vi "OEE_create_queues.vi"(8 "error_in":errorcluster, 11 "all_config_info_in":T1={"main_ini_file"={"SQL Driver"="", "SQL Server"="", "SQL Database"="", "SQL UID"="", "Reference table"="", "Reference history"="", "Archivisation CFG table"="", "Archivisation CFG history"="", "User table"="", "User history"="", "Default reference"="", "Update pulse[ms]"=0, "default language"="", "SCREEN 1 Left"=0, "SCREEN 1 Top"=10, "SCREEN 1 Width"=0, "SCREEN 1 Height"=0, "SCREEN 2 Left"=0, "SCREEN 2 Top"=0, "SCREEN 2 Width"=0, "SCREEN 2 Height"=10}, "SQL Password"="", "queue_refnums"={"MAIN_queue"=refnum, "SCREEN_1_queue"=refnum, "SCREEN_2_queue"=refnum, "PULSE_queue"=refnum, "GRAPH_TOGGLE_queue"=refnum}}) -> (0 "error_out":errorcluster, 3 "all_config_info_out":T1={"main_ini_file"={"SQL Driver"="", "SQL Server"="", "SQL Database"="", "SQL UID"="", "Reference table"="", "Reference history"="", "Archivisation CFG table"="", "Archivisation CFG history"="", "User table"="", "User history"="", "Default reference"="", "Update pulse[ms]"=0, "default language"="", "SCREEN 1 Left"=0, "SCREEN 1 Top"=10, "SCREEN 1 Width"=0, "SCREEN 1 Height"=0, "SCREEN 2 Left"=0, "SCREEN 2 Top"=0, "SCREEN 2 Width"=0, "SCREEN 2 Height"=10}, "SQL Password"="", "queue_refnums"={"MAIN_queue"=refnum, "SCREEN_1_queue"=refnum, "SCREEN_2_queue"=refnum, "PULSE_queue"=refnum, "GRAPH_TOGGLE_queue"=refnum}})   [LabVIEW 2019]
uses:
  ini/typedef/OEE_all_config_info.ctl
  ini/typedef/OEE_main_ini_file.ctl
  typedef/OEE_queue_refnums.ctl
  typedef/OEE_MAIN_queue_element.ctl
  MAIN/OEE_MAIN_sequence_state.ctl
  typedef/OEE_SCREEN_1_queue_element.ctl
  SCREEN_1/OEE_SCREEN_1_sequence_state.ctl
  typedef/OEE_SCREEN_2_queue_element.ctl
  SCREEN_2/OEE_SCREEN_2_sequence_state.ctl
  typedef/OEE_PULSE_queue_element.ctl
  PULSE/OEE_PULSE_sequence_state.ctl
  typedef/OEE_GRAPH_TOGGLE_TIMER_queue_element.ctl
  SCREEN_2/GRAPH_TOGGLE_TIMER/OEE_GRAPH_TOGGLE_TIMER_sequence_state.ctl
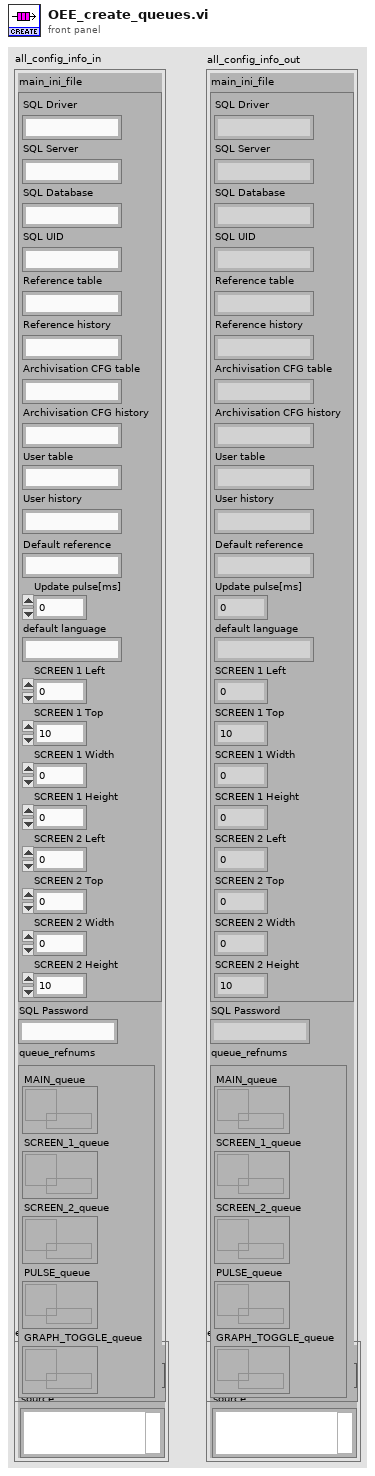
[diagram p1: front panel]
types:
  T1 = typedef "OEE_all_config_info.ctl" = cluster{"main_ini_file":T2, "SQL Password":string, "queue_refnums":T3}
  T2 = typedef "OEE_main_ini_file.ctl" = cluster{"SQL Driver":string, "SQL Server":string, "SQL Database":string, "SQL UID":string, "Reference table":string, "Reference history":string, "Archivisation CFG table":string, "Archivisation CFG history":string, "User table":string, "User history":string, "Default reference":string, "Update pulse[ms]":i32, "default language":string, "SCREEN 1 Left":i16, "SCREEN 1 Top":i16, "SCREEN 1 Width":i16, "SCREEN 1 Height":i16, "SCREEN 2 Left":i16, "SCREEN 2 Top":i16, "SCREEN 2 Width":i16, "SCREEN 2 Height":i16}
  T3 = typedef "OEE_queue_refnums.ctl" = cluster{"MAIN_queue":refnum<queue>, "SCREEN_1_queue":refnum<queue>, "SCREEN_2_queue":refnum<queue>, "PULSE_queue":refnum<queue>, "GRAPH_TOGGLE_queue":refnum<queue>}
  T4 = typedef "OEE_GRAPH_TOGGLE_TIMER_queue_element.ctl" = cluster{"state":T5, "variable":variant}
  T5 = typedef "OEE_GRAPH_TOGGLE_TIMER_sequence_state.ctl" = enum16{"initialize", "get_next_state", "start_toggling", "stop_toggling", "do_toggle", "error", "stop"}
  T6 = typedef "OEE_PULSE_queue_element.ctl" = cluster{"state":T7, "variable":variant}
  T7 = typedef "OEE_PULSE_sequence_state.ctl" = enum16{"initialize", "get_next_state", "start_pulses", "stop_pulses", "pulse", "error", "stop"}
  T8 = typedef "OEE_MAIN_queue_element.ctl" = cluster{"state":T9, "variable":variant}
  T9 = typedef "OEE_MAIN_sequence_state.ctl" = enum16{"initialize", "get_next_state", "get_SQL_data", "update_displays", "error", "stop"}
  T10 = typedef "OEE_SCREEN_2_queue_element.ctl" = cluster{"state":T11, "variable":variant}
  T11 = typedef "OEE_SCREEN_2_sequence_state.ctl" = enum16{"initialize", "get_next_state", "update", "show", "hide", "error", "stop"}
  T12 = typedef "OEE_SCREEN_1_queue_element.ctl" = cluster{"state":T13, "variable":variant}
  T13 = typedef "OEE_SCREEN_1_sequence_state.ctl" = enum16{"initialize", "get_next_state", "update", "show", "hide", "error", "stop"}
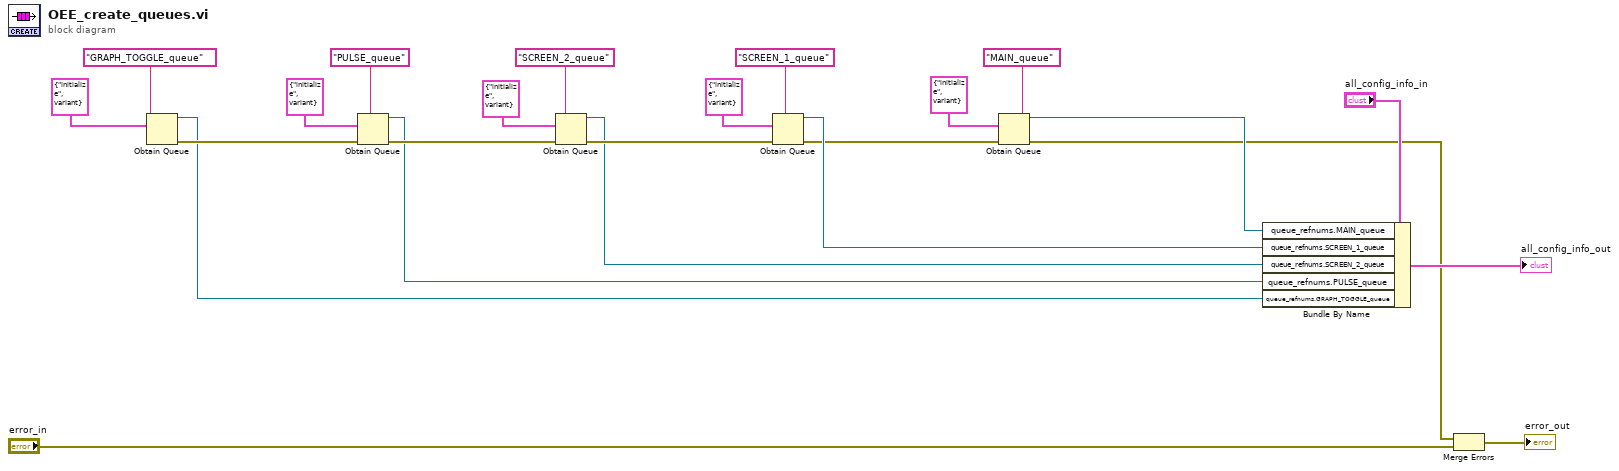
[diagram p0: block diagram]
diagram:
  n1 = Obtain Queue(name (unnamed)="GRAPH_TOGGLE_queue", element data type=T4 {"state"=enum."initialize", "variable"=variant} ("OEE_GRAPH_TOGGLE_TIMER_queue_element")) -> (queue out=w1:refnum<queue>, error out=w3:errorcluster)  [unwired: 3 in, 1 out]
  n2 = Obtain Queue(name (unnamed)="PULSE_queue", element data type=T6 {"state"=enum."initialize", "variable"=variant} ("SCANNER_queue_element"), error in (no error)=w3) -> (queue out=w5:refnum<queue>, error out=w6:errorcluster)  [unwired: 2 in, 1 out]
  n3 = Obtain Queue(name (unnamed)="SCREEN_2_queue", element data type=T10 {"state"=enum."initialize", "variable"=variant} ("SCANNER_queue_element"), error in (no error)=w6) -> (queue out=w14:refnum<queue>, error out=w19:errorcluster)  [unwired: 2 in, 1 out]
  n4 = Obtain Queue(name (unnamed)="SCREEN_1_queue", element data type=T12 {"state"=enum."initialize", "variable"=variant} ("OBJ_MAIN_queue_element"), error in (no error)=w19) -> (queue out=w15:refnum<queue>, error out=w11:errorcluster)  [unwired: 2 in, 1 out]
  n5 = Obtain Queue(name (unnamed)="MAIN_queue", element data type=T8 {"state"=enum."initialize", "variable"=variant} ("OBJ_MAIN_queue_element"), error in (no error)=w11) -> (queue out=w10:refnum<queue>, error out=w9:errorcluster)  [unwired: 2 in, 1 out]
  n6 = Bundle By Name(cluster="all_config_info_in", "queue_refnums.MAIN_queue"=w10, "queue_refnums.SCREEN_1_queue"=w15, "queue_refnums.SCREEN_2_queue"=w14, "queue_refnums.PULSE_queue"=w5, "queue_refnums.GRAPH_TOGGLE_queue"=w1) -> (→"all_config_info_out":T1)
  n7 = Merge Errors(w9, "error_in") -> (→"error_out":errorcluster)
